vi "Write Exception Status.vi"(7 "unit ID":u8, 8 "error in":errorcluster, 10 "exception status":u8 format="%02x", 11 "Modbus slave in":refnum<class "Modbus Slave.lvclass">) -> (0 "error out":errorcluster, 3 "Modbus slave out":refnum<class "Modbus Slave.lvclass">)   [LabVIEW 2013, in "Modbus Library - Advance.lvlib" / "Modbus Slave.lvclass"]
doc: "Sets the exception status stored in the device model."
uses:
  Modbus Slave.lvclass
  Modbus Slave.lvclass/Modbus Slave.ctl
  Standard Data Model/Standard Data Model.lvclass
  Super Data Model/Super Data Model.lvclass
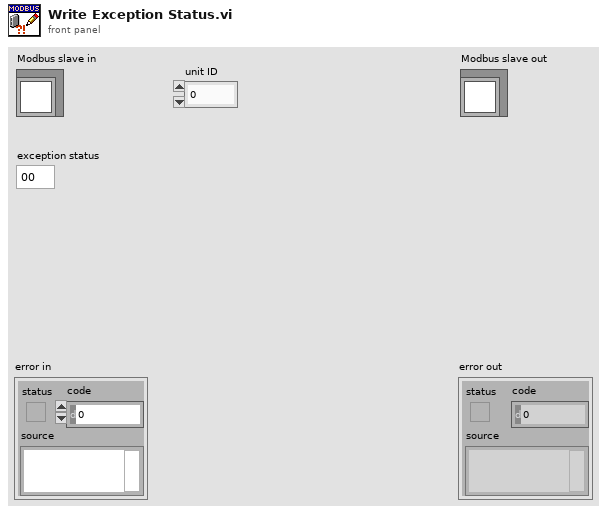
[diagram p1: front panel]
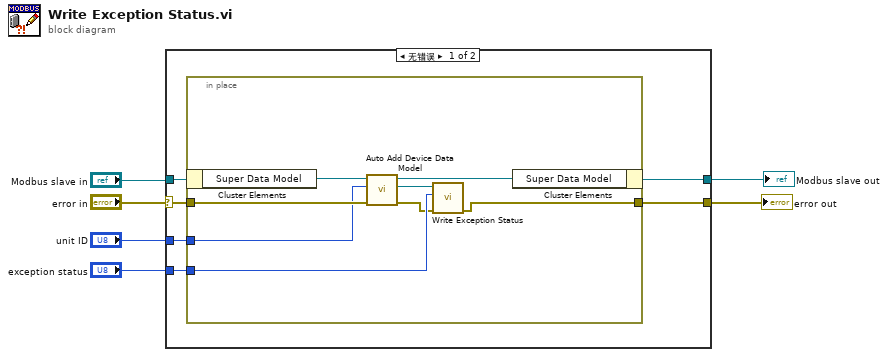
[diagram p0: block diagram]
diagram:
  n1 = case shown="无错误" "error in" {
    selector: "error in" -> [w12 w22]
    tunnel: "unit ID" -> [w11 _]
    tunnel: "Modbus slave in" -> [w10 w21]
    tunnel: [w9 w21] -> w2
    tunnel: [w8 w22] -> w1
    tunnel: "exception status" -> [w7 _]
    frame No Error {
      n2 = in-place {
        in-place-border: w12 -> [w18]
        in-place-border: [w20] -> w8
        in-place-border: w11 -> [w17]
        in-place-border: w7 -> [w16]
        n3 = in-place-cluster #1(w10) -> ("Super Data Model"=w19:refnum<class "Super Data Model.lvclass">)
        n4 = call "Auto Add Device Data Model.vi"("error in"=w18, "unit ID"=w17, "Super Data Model in"=w19) -> ("error out"=w15:errorcluster, "device data model"=w13:refnum<class "Standard Data Model.lvclass">, "Super Data Model out"=w14:refnum<class "Super Data Model.lvclass">)  [unwired: 6 in]
        n5 = call-dynamic "Write Exception Status.vi"("error in"=w15, "exception status"=w16, "device data model in"=w13) -> ("error out"=w20:errorcluster)  [unwired: 7 in, 1 out]
        n6 = in-place-cluster #1("Super Data Model"=w14) -> (w9:refnum<class "Modbus Slave.lvclass">)
      }
    }
    frame Error {
    }
  }
  "Modbus slave out" <- w2
  "error out" <- w1
